vi "ERIO LCD Write.vi"(6 "Amplitude":dbl, 7 "error in (no error)":errorcluster, 8 "Stage Number":string="Stage 1", 9 "Current Pos > Threshold?":bool, 10 "Character LCD in":refnum<class "Character LCD.lvclass">) -> (0 "error out":errorcluster, 3 "LCD out":refnum<class "Character LCD.lvclass">)   [LabVIEW 2017]
doc: "This VI manages writing to the LCD, during normal operation the current amplitude value will appear, once the encoder position has covered an entire stage, write 'Stage # Complete' for one second.\n\nORIGINAL CODE: \nBy: National Instruments\n NI LabVIEW RIO Evaluation Kit\n Code example \"5- Startup Application\"\n www.ni.com/embeddedsystems\n\nUPDATED CODE: Adds NI SystemLink and NI AWS LabVIEW Tookit functionality for demonstration. \nBy: James Tillett\n Endeavor Engineering Inc.\n www.endeavoreng.com"
uses:
  EmbeddedDisplay/Hitachi HD44780/Host/Internal/LCD Class/Character LCD.lvclass
  EmbeddedDisplay/Hitachi HD44780/Common/Control/cursor position.ctl
  EmbeddedDisplay/Hitachi HD44780/Host/Public/Output (String).vi
  EmbeddedDisplay/Hitachi HD44780/Common/HD44780 Common.lvlib
  EmbeddedDisplay/Hitachi HD44780/Host/HD44780 Host.lvlib
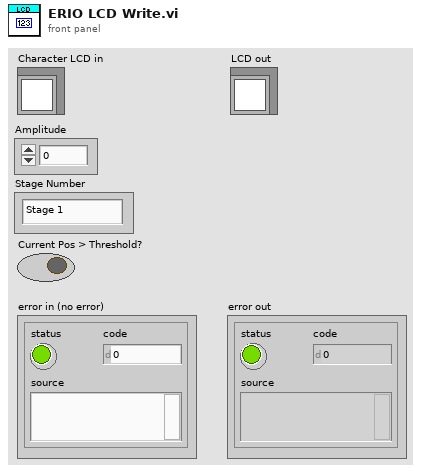
[diagram p1: front panel]
types:
  T1 = typedef "HD44780 Common.lvlib/cursor position.ctl" = cluster{"row":i8, "column":i8}
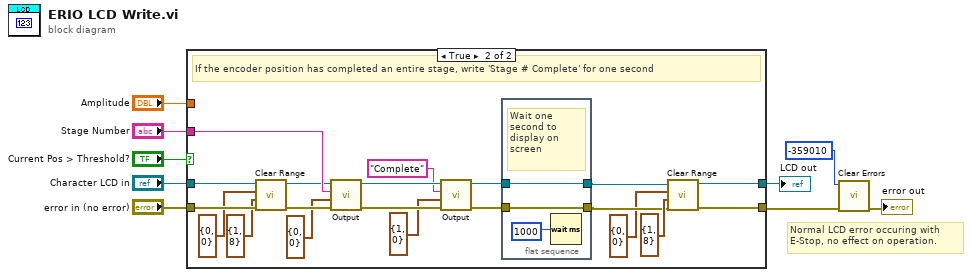
[diagram p0: block diagram]
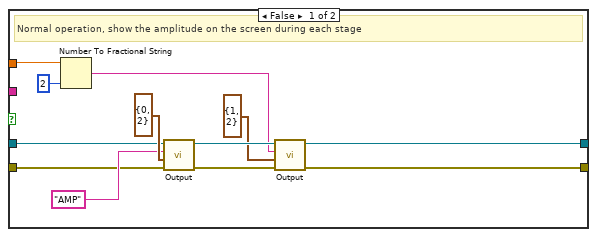
[diagram p2: hidden frame]
diagram:
  # "Normal LCD error occuring with \nE-Stop, no effect on operation."
  n1 = case shown="True" "Current Pos > Threshold?" {
    tunnel: "error in (no error)" -> [w15 w27]
    tunnel: "Character LCD in" -> [w16 w29]
    tunnel: [w14 w32] -> w2
    tunnel: [w13 w31] -> w3
    tunnel: "Stage Number" -> [_ w38]
    tunnel: "Amplitude" -> [w11 _]
    frame False {
      # "Normal operation, show the amplitude on the screen during each stage"
      n2 = Number To Fractional String(number=w11, precision (6)=i16 2) -> (F-format string=w10:string)  [unwired: 2 in]
      n3 = call-poly "Output.vi"("error in (no error)"=w15, "position"=T1 {"row"=0, "column"=2}, "text"="AMP", "LCD in"=w16) -> ("error out"=w20:errorcluster, "LCD out"=w21:refnum<class "Character LCD.lvclass">)  [unwired: 5 in, 1 out]
      n4 = call-poly "Output.vi"("error in (no error)"=w20, "position"=T1 {"row"=1, "column"=2}, "text"=w10, "LCD in"=w21) -> ("error out"=w13:errorcluster, "LCD out"=w14:refnum<class "Character LCD.lvclass">)  [unwired: 5 in, 1 out]
    }
    frame True {
      # "If the encoder position has completed an entire stage, write 'Stage # Complete' for one second"
      n5 = call "Clear Range.vi"("error in (no error)"=w27, "end position (end of line)"=cluster{"row":i8, "column":i8} {"row"=1, "column"=8} ("start position"), "start position"=cluster{"row":i8, "column":i8} {"row"=0, "column"=0}, "LCD in"=w29) -> ("error out"=w26:errorcluster, "LCD out"=w28:refnum<class "Character LCD.lvclass">)  [unwired: 6 in]
      n6 = call-poly "Output.vi"("error in (no error)"=w26, "position"=cluster{"row":i8, "column":i8} {"row"=0, "column"=0} ("start position"), "text"=w38, "LCD in"=w28) -> ("error out"=w41:errorcluster, "LCD out"=w40:refnum<class "Character LCD.lvclass">)  [unwired: 5 in, 1 out]
      n7 = call-poly "Output.vi"("error in (no error)"=w41, "position"=cluster{"row":i8, "column":i8} {"row"=1, "column"=0} ("start position"), "text"="Complete", "LCD in"=w40) -> ("error out"=w37:errorcluster, "LCD out"=w36:refnum<class "Character LCD.lvclass">)  [unwired: 5 in, 1 out]
      n8 = flat-sequence {
        tunnel: w37 -> [w43]
        tunnel: [w43] -> w33
        tunnel: w36 -> [w42]
        tunnel: [w42] -> w34
        frame #0 {
          # "Wait one second to display on screen"
          n9 = Wait (ms)(milliseconds to wait=u32 1000) -> ()  [unwired: 1 out]
        }
      }
      n10 = call "Clear Range.vi"("error in (no error)"=w33, "end position (end of line)"=cluster{"row":i8, "column":i8} {"row"=1, "column"=8} ("start position"), "start position"=cluster{"row":i8, "column":i8} {"row"=0, "column"=0}, "LCD in"=w34) -> ("error out"=w31:errorcluster, "LCD out"=w32:refnum<class "Character LCD.lvclass">)  [unwired: 6 in]
    }
  }
  "LCD out" <- w2
  n11 = call <vilib>:"Clear Errors.vi"("error in (no error)"=w3, "specific error code to clear (0: all)"=-359010) -> ("error out"=→"error out":errorcluster)  [unwired: 4 in, 1 out]
